vi "ArgHandler.vi"() -> ()   [LabVIEW 2019]
panel:
  out "error out":errorcluster
  out "arguments":string[](array[string])
  out "application name":string
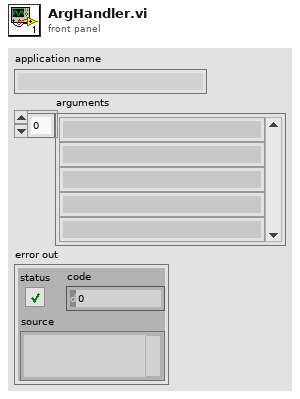
[diagram p1: front panel]
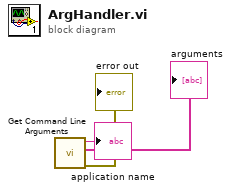
[diagram p0: block diagram]
diagram:
  n1 = call <vilib>:"Get Command Line Arguments.vi"() -> ("error out"=→"error out":errorcluster, "arguments"=→"arguments":string[], "application name"=→"application name":string)  [unwired: 9 in]
